vi "subvi_Get Folder Hierarchy.vi"(7 "Hierarchy":T1 items=["root", "1", "2", "3"], 8 "error in (no error)":errorcluster, 11 "Path":path) -> (0 "error out":errorcluster, 2 "appended array":string[](array[string]), 3 "Path Array":path[](array[path]))   [LabVIEW 2015, in "File Version Lib.lvlib"]
uses:
  File Version Lib.lvlib
  control_Hierarchy.ctl
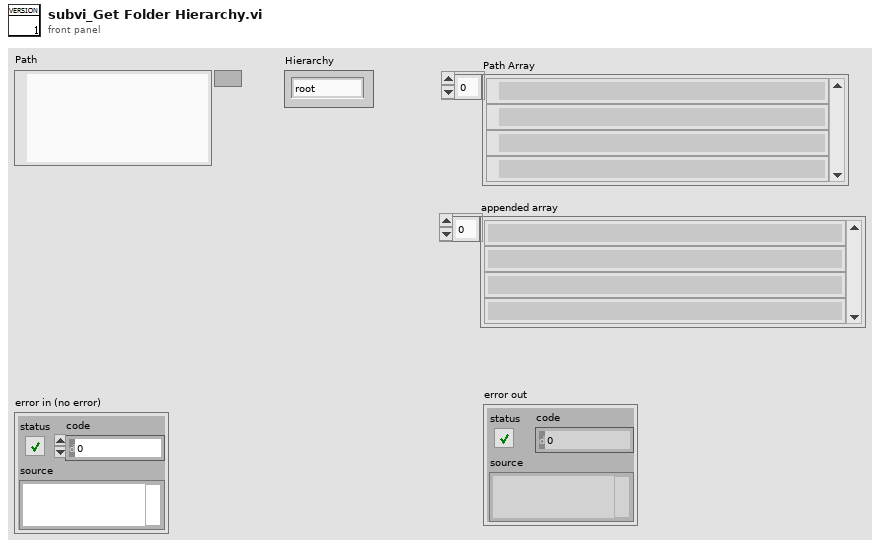
[diagram p1: front panel]
types:
  T1 = typedef "File Version Lib.lvlib/control_Hierarchy.ctl" = u16
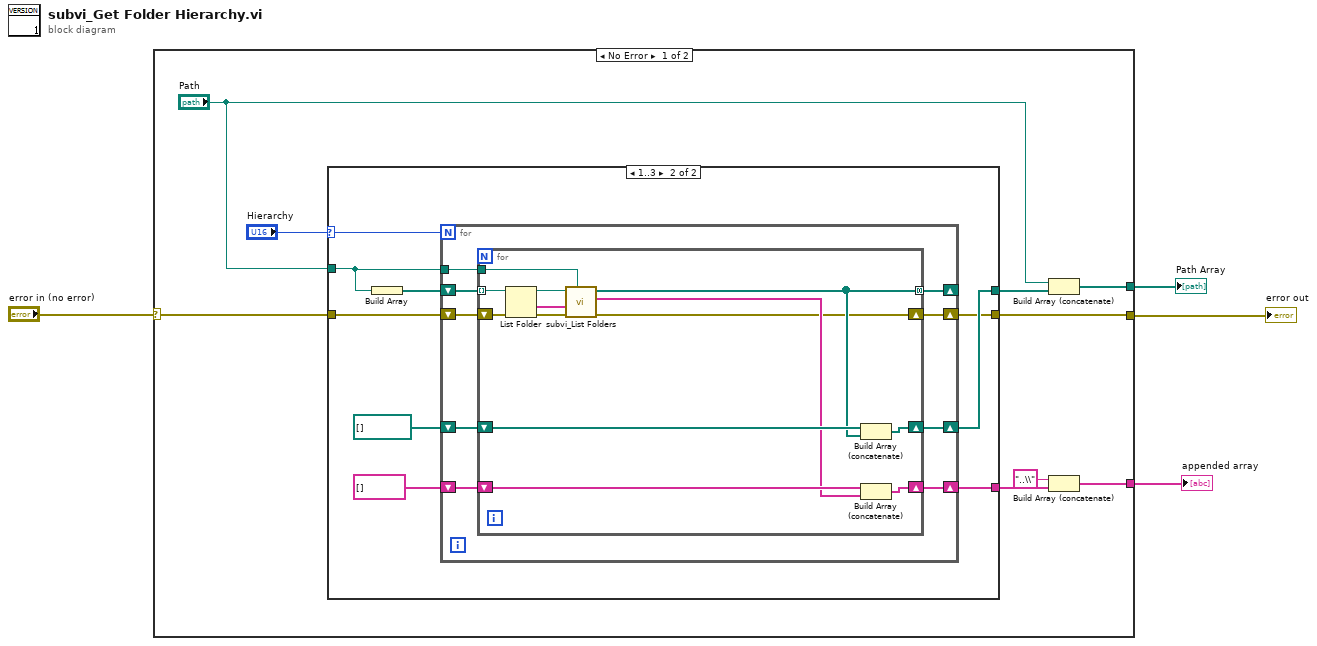
[diagram p0: block diagram]
diagram:
  n1 = case shown="No Error" "error in (no error)" {
    selector: "error in (no error)" -> [w6 w46]
    tunnel: [w10 _] -> w4
    tunnel: [w7 _] -> w3
    tunnel: [w5 w46] -> w1
    frame No Error {
      n2 = case shown="1..3" "Hierarchy" {
        selector: "Hierarchy" -> [_ w23]
        tunnel: "Path" -> [_ w15]
        tunnel: [_ w20] -> w12
        tunnel: [_ w18] -> w9
        tunnel: [w14 w17] -> w5
        tunnel: w6 -> [w14 w16]
        frame 0, Default {
        }
        frame 1..3 {
          n3 = Build Array(w15) -> (w21:path[])
          n4 = for {
            N: w23 -> [_]
            shift-right: [w29] -> w20
            shift-left: path[] [] -> [w30]
            shift-right: [w31] -> _
            shift-left: w21 -> [w32]
            shift-right: [w28] -> w18
            shift-left: string[] [] -> [w27]
            shift-right: [w26] -> w17
            shift-left: w16 -> [w25]
            tunnel: w15 -> [w24]
            n5 = for {
              tunnel: w32 -> [w45] mode=indexing
              tunnel: [w37] -> w31 mode=concatenating
              shift-right: [w43] -> w29
              shift-left: w30 -> [w44]
              shift-right: [w42] -> w28
              shift-left: w27 -> [w41]
              shift-right: [w35] -> w26
              shift-left: w25 -> [w34]
              tunnel: w24 -> [w33]
              n6 = List Folder(path=w45, error in=w34) -> (path out=w40:path, folder names=w39:string[], error out=w38:errorcluster)  [unwired: 2 in, 1 out]
              n7 = call "subvi_List Folders.vi"("root path"=w33, "error in (no error)"=w38, "folder names"=w39, "path"=w40) -> ("error out"=w35:errorcluster, "Path Strings"=w36:string[], "Paths"=w37:path[])  [unwired: 5 in]
              n8 = Build Array (concatenate)(w44, w37) -> (w43:path[])
              n9 = Build Array (concatenate)(w41, w36) -> (w42:string[])
            }
          }
        }
      }
      n10 = Build Array (concatenate)("Path", w12) -> (w10:path[])
      n11 = Build Array (concatenate)("..\\", w9) -> (w7:string[])
    }
    frame Error {
    }
  }
  "Path Array" <- w4
  "appended array" <- w3
  "error out" <- w1
